vi "TMP007 Init.vi"(7 "I2C Channel":u8=1, 8 "error in (no error)":errorcluster, 9 "Samples to Average":u16(ring) items=["1 sample, .26s conversion"=0, "2 samples, .51s conversion"=512, "4 samples, 1.01s conversion"=1024, "8 samples, 2.01s conversion"=1536, "16 samples, 4.01s conversion"=2048], 10 "I2C Slave Address":u8=64 format="%.0x", 11 "LINX Resource in":T1) -> (0 "error out":errorcluster, 3 "LINX Resource out":T1)   [LabVIEW 2014]
uses:
  <vilib>/MakerHub/LINX/Private/Type Defs/LINX Ref.ctl
  <vilib>/MakerHub/LINX/Private/Type Defs/Platform.ctl
  <vilib>/MakerHub/LINX/Private/Type Defs/Interface.ctl
  <vilib>/MakerHub/LINX/Private/Device/Type Defs/LINX Device Config.ctl
  <vilib>/MakerHub/LINX/Private/Device/Type Defs/TCP Config.ctl
  <vilib>/MakerHub/LINX/Private/Device/Type Defs/Channels.ctl
  <vilib>/MakerHub/LINX/LMH-LINX.lvlib
  <vilib>/MakerHub/LINX/Private/Device/Device.lvlib
panel:
  # "Each sample takes .25s to convert\nThere are some other conversion modes that include idle times, but I didn't include those modes"
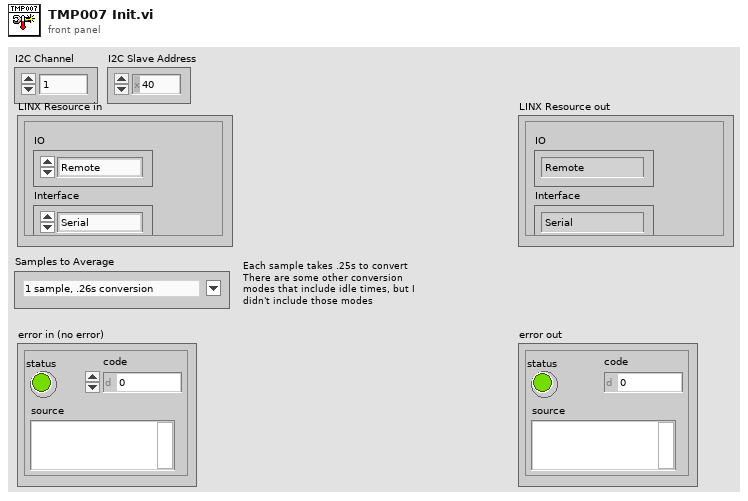
[diagram p1: front panel]
types:
  T1 = typedef "LMH-LINX.lvlib/LINX Ref.ctl" = cluster{"IO":T2, "Interface":T3, "LINX Device Config":T4}
  T2 = typedef "LMH-LINX.lvlib/Platform.ctl" = enum16{"Remote", "Local"}
  T3 = typedef "LMH-LINX.lvlib/Interface.ctl" = enum16{"Serial", "TCP"}
  T4 = typedef "LMH-LINX.lvlib/Device.lvlib/LINX Device Config.ctl" = cluster{"Interface":T3, "COM Port":refnum<visa-resource-name>, "TCP Configuration":T5, "Device Family":u8, "Device ID":u8, "Device Name":string, "TCP Ref":refnum<k5>, "Channels":T6}
  T5 = typedef "LMH-LINX.lvlib/Device.lvlib/TCP Config.ctl" = cluster{"IP Address":string, "Port":u16}
  T6 = typedef "LMH-LINX.lvlib/Channels.ctl" = cluster{"DI":u8[], "DO":u8[], "AI":u8[], "AO":u8[], "PWM":u8[], "QE":u8[], "UART":u8[], "I2C 2":u8[], "SPI":u8[], "CAN":u8[], "Servo":u8[], "AI Ref (V)":dbl, "AI Resolution (Bits)":u8, "AO Ref (V)":dbl, "AO Resolution (Bits)":u8}
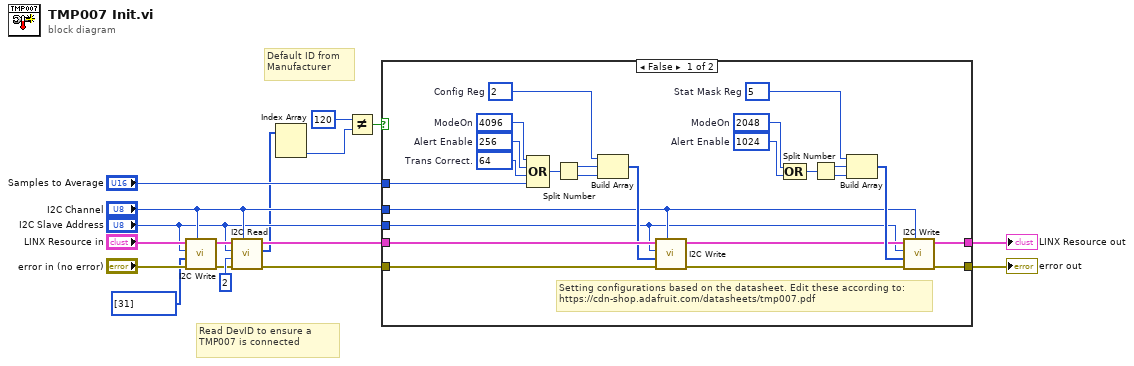
[diagram p0: block diagram]
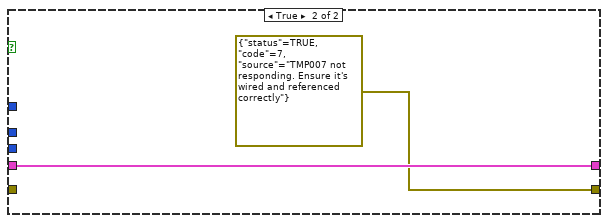
[diagram p2: hidden frame]
diagram:
  # "Default ID from Manufacturer"
  # "Read DevID to ensure a TMP007 is connected"
  n1 = call <vilib>:"I2C Write.vi"("I2C Channel"="I2C Channel", "Error In"="error in (no error)", "Data"=u8[] [31], "I2C Slave Address (0)"="I2C Slave Address", "LINX Resource"="LINX Resource in") -> ("Error Out"=w10:errorcluster, "LINX Resource"=w9:T1)  [unwired: 5 in]
  n2 = call <vilib>:"I2C Read.vi"("I2C Channel"="I2C Channel", "Error In"=w10, "Bytes To Read"=u8 2, "I2C Slave Address (0)"="I2C Slave Address", "LINX Resource"=w9) -> ("Error Out"=w13:errorcluster, "Data"=w3:u8[], "LINX Resource"=w14:T1)  [unwired: 4 in]
  n3 = Index Array(array=w3) -> (element #2=w1:u8)  [unwired: 2 in, 1 out]
  n4 = Not Equal?(x=u8 120, y=w1) -> (x != y?=w7:bool)
  n5 = case shown="False" w7 {
    tunnel: w14 -> [w41 w43]
    tunnel: [w19 w43] -> w16
    tunnel: w13 -> [w40 _]
    tunnel: [w18 errorcluster {"status"=TRUE, "code"=7, "source"="TMP007 not responding. Ensure it's wired and referenced correctly"} ("error constant")] -> w15
    tunnel: "Samples to Average" -> [w39 _]
    tunnel: "I2C Channel" -> [w21 _]
    tunnel: "I2C Slave Address" -> [w20 _]
    frame False {
      w30 = u8 5  # Stat Mask Reg
      w25 = u16 1024  # Alert Enable
      w26 = u16 2048  # ModeOn
      w32 = u8 2  # Config Reg
      w38 = u16 64  # Trans Correct.
      w37 = u16 256  # Alert Enable
      w36 = u16 4096  # ModeOn
      # "Setting configurations based on the datasheet. Edit these according to:\nhttps://cdn-shop.adafruit.com/datasheets/tmp007.pdf"
      n6 = Compound Arithmetic op=OR(w36, w37, w38, w39) -> (w35:u16)
      n7 = Split Number(x=w35) -> (hi(x)=w34:u8, lo(x)=w33:u8)
      n8 = Build Array(w32, w34, w33) -> (w31:u8[])
      n9 = call <vilib>:"I2C Write.vi"("I2C Channel"=w21, "Error In"=w40, "Data"=w31, "I2C Slave Address (0)"=w20, "LINX Resource"=w41) -> ("Error Out"=w22:errorcluster, "LINX Resource"=w23:T1)  [unwired: 5 in]
      n10 = Compound Arithmetic op=OR(w26, w25) -> (w27:u16)
      n11 = Split Number(x=w27) -> (hi(x)=w28:u8, lo(x)=w29:u8)
      n12 = Build Array(w30, w28, w29) -> (w24:u8[])
      n13 = call <vilib>:"I2C Write.vi"("I2C Channel"=w21, "Error In"=w22, "Data"=w24, "I2C Slave Address (0)"=w20, "LINX Resource"=w23) -> ("Error Out"=w18:errorcluster, "LINX Resource"=w19:T1)  [unwired: 5 in]
    }
    frame True {
    }
  }
  "error out" <- w15
  "LINX Resource out" <- w16
